vi "Find_usb_com_port_number.vi"(6 "Search key for all output":string, 8 "error in (no error)":errorcluster, 9 "Use this string instead":string, 10 "Pid":string, 11 "Vid":string) -> (0 "error out":errorcluster, 1 "Created search key":string, 2 "Found com port":bool, 3 "Comport":string, 4 "Devcon output":string="No matching devices found.\r\n", 5 "Com port number":string)   [LabVIEW 2013]
panel:
  in  "USB search key":string="USB\\VID_1BC7*PID_1010*MI_02* "
  # "usb\\vid_1bc7*pid_1010*MI_03*"
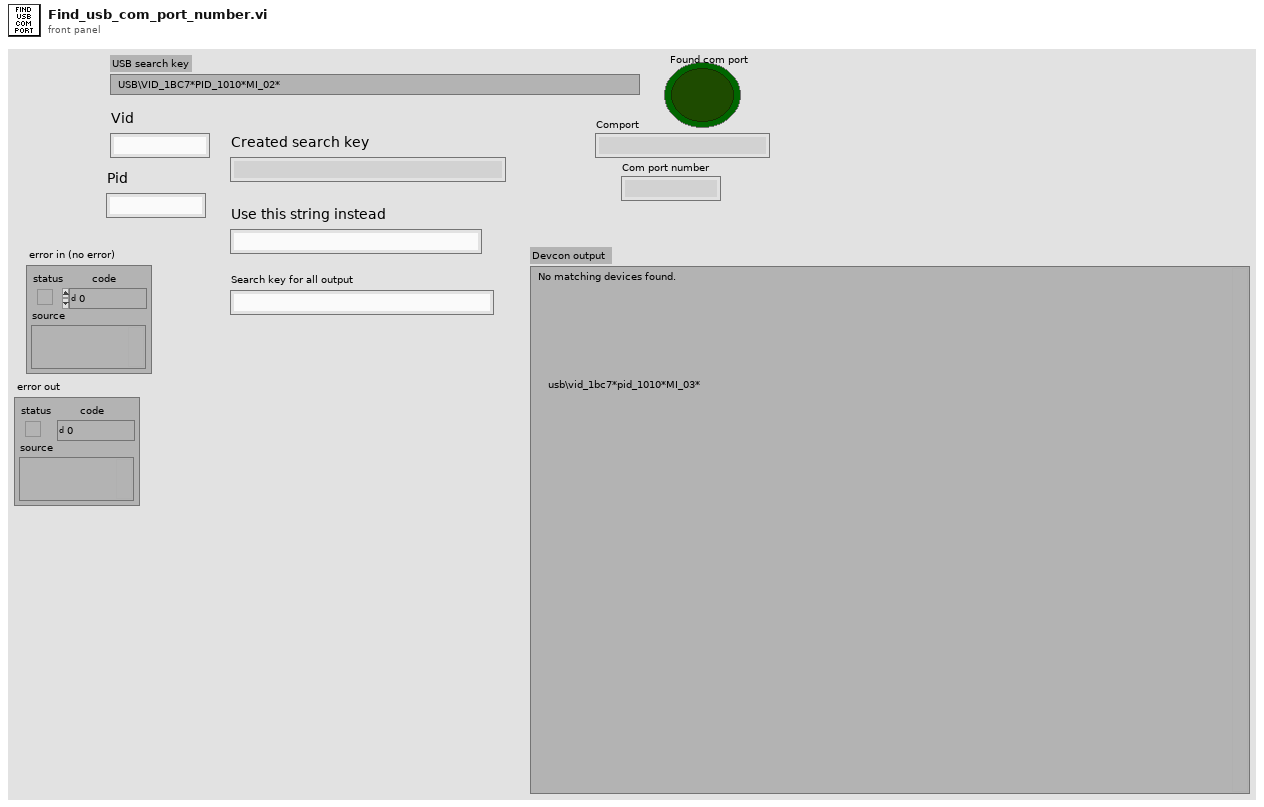
[diagram p1: front panel]
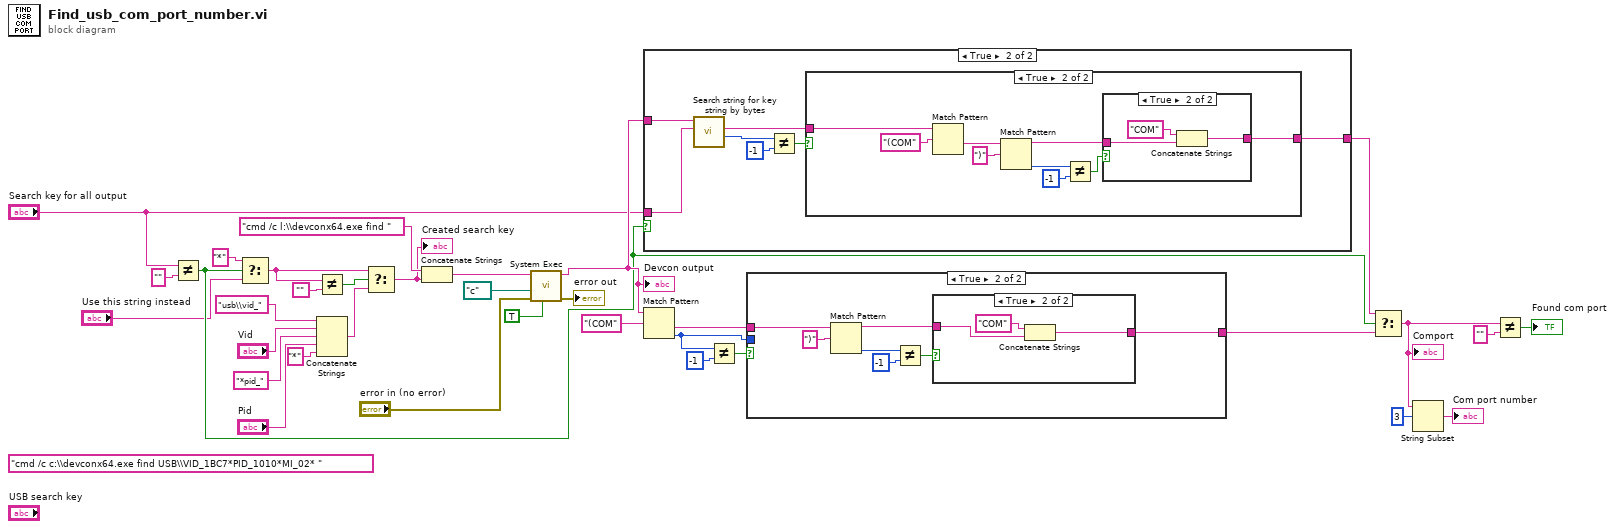
[diagram p0: block diagram]
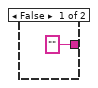
[diagram p2: hidden frame]
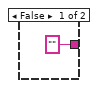
[diagram p3: hidden frame]
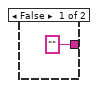
[diagram p4: hidden frame]
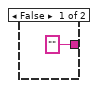
[diagram p5: hidden frame]
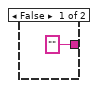
[diagram p6: hidden frame]
diagram:
  (unwired) "cmd /c c:\\devconx64.exe find USB\\VID_1BC7*PID_1010*MI_02* " ("command line")
  n1 = Not Equal?(x="Search key for all output", y="") -> (x != y?=w7:bool)
  n2 = Select(t="*", s=w7, f="Use this string instead") -> (s? t:f=w4:string)
  n3 = Not Equal?(x=w4, y="") -> (x != y?=w15:bool)
  n4 = Concatenate Strings("usb\\vid_" ("string"), "Vid", "*pid_" ("string"), "Pid", "*" ("string")) -> (w14:string)
  n5 = Select(t=w4, s=w15, f=w14) -> (s? t:f=w13:string)
  "Created search key" <- w13
  n6 = Concatenate Strings("cmd /c l:\\devconx64.exe find ", w13) -> (w24:string)
  n7 = call <vilib>:"System Exec.vi"("run minimized? (F)"=TRUE, "error in (no error)"="error in (no error)", "working directory"=path "c:/", "command line"=w24) -> ("error out"=→"error out":errorcluster, "standard output"=w11:string)  [unwired: 4 in, 2 out]
  "Devcon output" <- w11
  n8 = case shown="True" w7 {
    tunnel: w11 -> [_ w39]
    tunnel: "Search key for all output" -> [_ w38]
    tunnel: ["" ("standard output") w40] -> w9
    frame False {
    }
    frame True {
      n9 = call "Search string for key string by bytes.vi"("Search for string"=w38, "String"=w39) -> ("Offset past match"=w36:i32, "After"=w37:string)  [unwired: 5 in, 3 out]
      n10 = Not Equal?(x=w36, y=-1) -> (x != y?=w41:bool)
      n11 = case shown="True" w41 {
        tunnel: w37 -> [_ w51]
        tunnel: ["" ("standard output") w44] -> w40
        frame False {
        }
        frame True {
          n12 = Match Pattern(string=w51, regular expression="(COM") -> (after substring=w49:string)  [unwired: 1 in, 3 out]
          n13 = Match Pattern(string=w49, regular expression=")") -> (before substring=w46:string, offset past match=w45:i32)  [unwired: 1 in, 2 out]
          n14 = Not Equal?(x=w45, y=-1) -> (x != y?=w48:bool)
          n15 = case shown="True" w48 {
            tunnel: ["" ("standard output") w54] -> w44
            tunnel: w46 -> [_ w55]
            frame False {
            }
            frame True {
              n16 = Concatenate Strings("COM" ("string"), w55) -> (w54:string)
            }
          }
        }
      }
    }
  }
  n17 = Match Pattern(string=w11, regular expression="(COM") -> (after substring=w26:string, offset past match=w27:i32)  [unwired: 1 in, 2 out]
  n18 = Not Equal?(x=w27, y=-1) -> (x != y?=w28:bool)
  n19 = case shown="True" w28 {
    tunnel: w27 -> [_ _]
    tunnel: w26 -> [_ w60]
    tunnel: ["" ("standard output") w58] -> w8
    frame False {
    }
    frame True {
      n20 = Match Pattern(string=w60, regular expression=")") -> (before substring=w59:string, offset past match=w62:i32)  [unwired: 1 in, 2 out]
      n21 = Not Equal?(x=w62, y=-1) -> (x != y?=w61:bool)
      n22 = case shown="True" w61 {
        tunnel: ["" ("standard output") w66] -> w58
        tunnel: w59 -> [_ w67]
        frame False {
        }
        frame True {
          n23 = Concatenate Strings("COM" ("string"), w67) -> (w66:string)
        }
      }
    }
  }
  n24 = Select(t=w9, s=w7, f=w8) -> (s? t:f=w3:string)
  "Comport" <- w3
  n25 = String Subset(string=w3, offset (0)=3) -> (substring=→"Com port number":string)  [unwired: 1 in]
  n26 = Not Equal?(x=w3, y="") -> (x != y?=→"Found com port":bool)
